vi "ReadAndParse.vi"(8 "error in (no error)":errorcluster, 11 "Path":path) -> (0 "error out":errorcluster, 3 "Config":T1)   [LabVIEW 2020]
uses:
  <vilib>/WebServerConfig/Config.ctl
  <vilib>/WebServerConfig/Server.ctl
  <vilib>/WebServerConfig/Alias.ctl
  <vilib>/WebServerConfig/ErrorDocument.ctl
  <vilib>/WebServerConfig/Action.ctl
  <vilib>/WebServerConfig/Redirect.ctl
  <vilib>/WebServerConfig/Interface.ctl
  <vilib>/WebServerConfig/AddHandler.ctl
  <vilib>/WebServerConfig/SSL.ctl
  <vilib>/WebServerConfig/CustomLog.ctl
  <vilib>/WebServerConfig/LoadModule.ctl
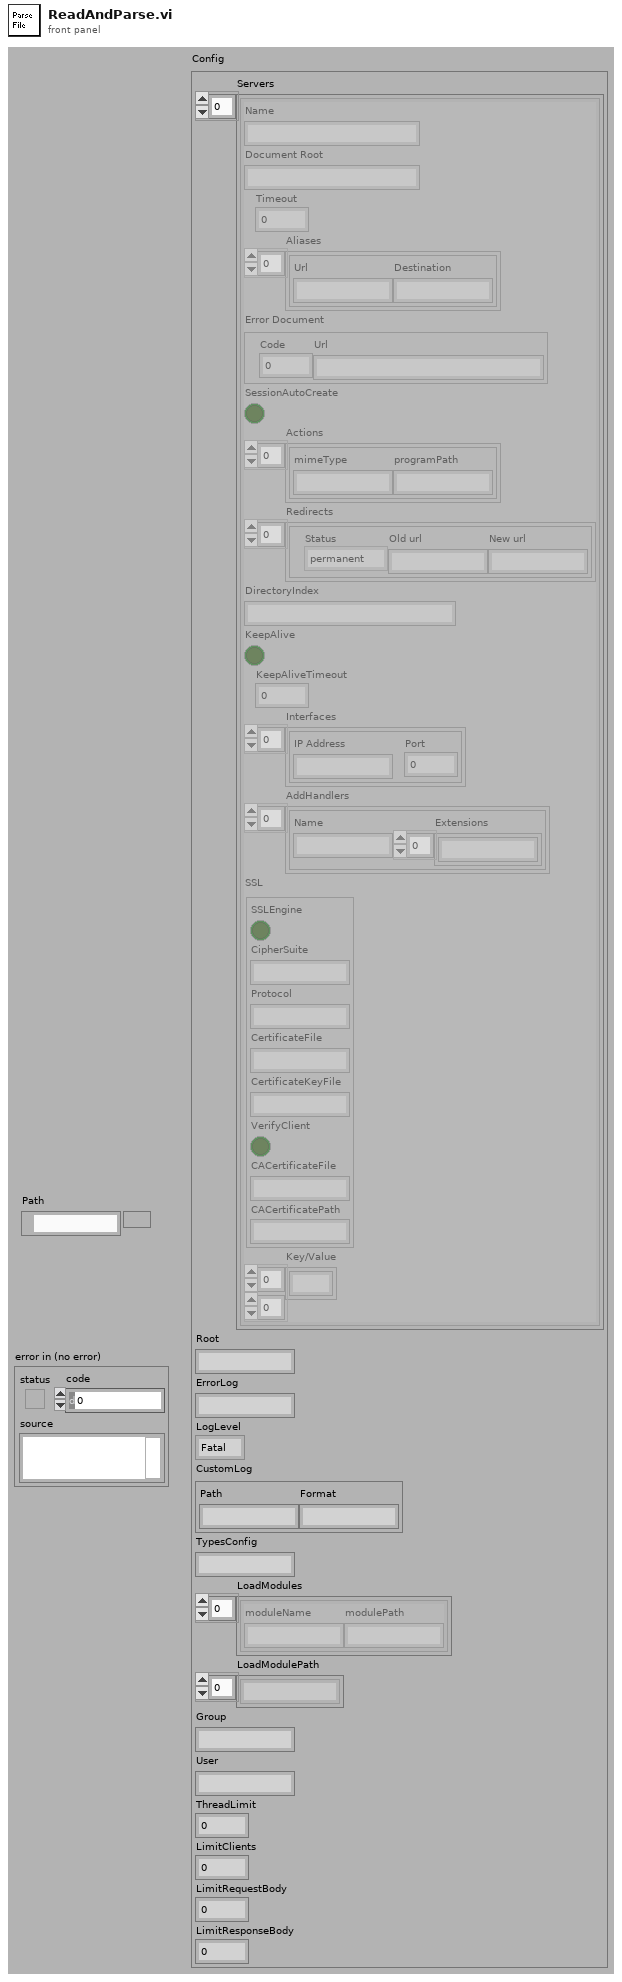
[diagram p1: front panel]
types:
  T1 = typedef "Config.ctl" = cluster{"Servers":T2[], "Root":string, "ErrorLog":string, "LogLevel":enum16{"Fatal", "Error", "Warn", "Info", "Debug", "5", "6", "7", "8", "Verbose"}, "CustomLog":T10, "TypesConfig":string, "LoadModules":T11[], "LoadModulePath":string[], "Group":string, "User":string, "ThreadLimit":u32, "LimitClients":u32, "LimitRequestBody":u32, "LimitResponseBody":u32}
  T2 = typedef "Server.ctl" = cluster{"Name":string, "Document Root":string, "Timeout":u32, "Aliases":T3[], "Error Document":T4, "SessionAutoCreate":bool, "Actions":T5[], "Redirects":T6[], "DirectoryIndex":string, "KeepAlive":bool, "KeepAliveTimeout":u32, "Interfaces":T7[], "AddHandlers":T8[], "SSL":T9, "Key/Value":string[][]}
  T3 = typedef "Alias.ctl" = cluster{"Url":string, "Destination":string}
  T4 = typedef "ErrorDocument.ctl" = cluster{"Code":u16, "Url":string}
  T5 = typedef "Action.ctl" = cluster{"mimeType":string, "programPath":string}
  T6 = typedef "Redirect.ctl" = cluster{"Status":enum16{"permanent", "temp", "seeother", "gone"}, "Old url":string, "New url":string}
  T7 = typedef "Interface.ctl" = cluster{"IP Address":string, "Port":u16}
  T8 = typedef "AddHandler.ctl" = cluster{"Name":string, "Extensions":string[]}
  T9 = typedef "SSL.ctl" = cluster{"SSLEngine":bool, "CipherSuite":string, "Protocol":string, "CertificateFile":string, "CertificateKeyFile":string, "VerifyClient":bool, "CACertificateFile":string, "CACertificatePath":string}
  T10 = typedef "CustomLog.ctl" = cluster{"Path":string, "Format":string}
  T11 = typedef "LoadModule.ctl" = cluster{"moduleName":string, "modulePath":string}
  T12 = enum16{"open", "replace", "create", "open or create", "replace or create", "replace or create with confirmation"}
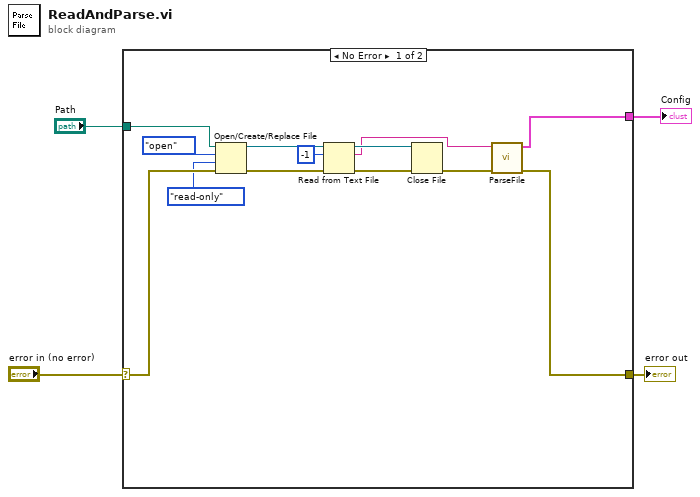
[diagram p0: block diagram]
diagram:
  n1 = case shown="No Error" "error in (no error)" {
    selector: "error in (no error)" -> [w14 w18]
    tunnel: [w13 w18] -> w3
    tunnel: "Path" -> [w8 _]
    tunnel: [w5 _] -> w1
    frame No Error {
      n2 = Open/Create/Replace File(file path (use dialog)=w8, error in=w14, operation (0:open)=T12."open", access (0:read/write)=enum16{"read/write", "read-only", "write-only"}."read-only") -> (refnum out=w12:refnum<file>, error out=w17:errorcluster)  [unwired: 2 in, 1 out]
      n3 = Read from Text File(file (use dialog)=w12, count=-1, error in=w17) -> (refnum out=w11:refnum<file>, text=w10:string, error out=w16:errorcluster)  [unwired: 1 in, 1 out]
      n4 = Close File(refnum=w11, error in=w16) -> (error out=w15:errorcluster)  [unwired: 1 out]
      n5 = call <vilib>:"ParseFile.vi"("error in (no error)"=w15, "FileContents"=w10) -> ("error out"=w13:errorcluster, "Config"=w5:T1)  [unwired: 8 in]
    }
    frame Error {
    }
  }
  "Config" <- w1
  "error out" <- w3
